vi "Read UI Refnum.vi"(8 "error in (no error)":errorcluster, 11 "SerializableObject in":refnum<class "SerializableObject.lvclass">) -> (0 "error out":errorcluster, 2 "VI Refnum":refnum<vi>, 3 "SerializableObject out":refnum<class "SerializableObject.lvclass">)   [LabVIEW 2015, in "SerializableObject.lvclass"]
uses:
  SerializableObject.lvclass
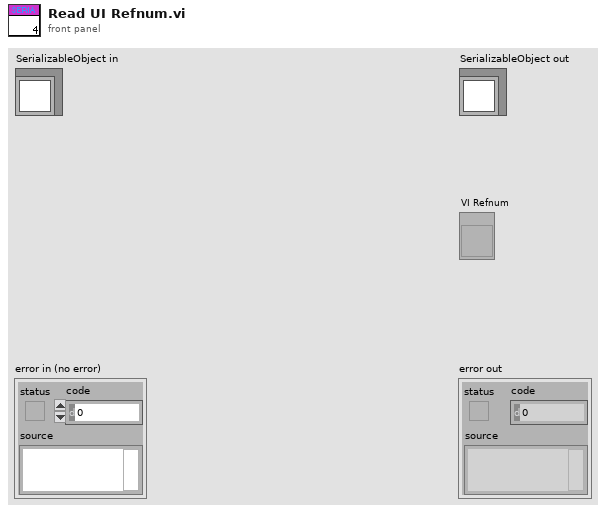
[diagram p1: front panel]
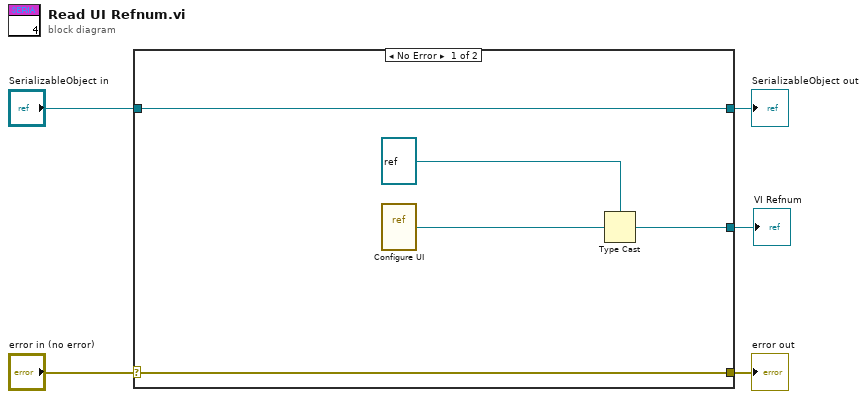
[diagram p0: block diagram]
diagram:
  n1 = case shown="No Error" "error in (no error)" {
    selector: "error in (no error)" -> [w9 w12]
    tunnel: [w9 w12] -> w4
    tunnel: [w10 w11] -> w2
    tunnel: "SerializableObject in" -> [w10 w11]
    tunnel: [w6 _] -> w1
    frame No Error {
      n2 = vi-ref "Configure UI.vi"() -> (w8:refnum<vi>)
      n3 = Type Cast(type=refnum<vi> refnum ("vi reference"), x=w8) -> (*(type *) &x=w6:refnum<vi>)
    }
    frame Error {
    }
  }
  "error out" <- w4
  "SerializableObject out" <- w2
  "VI Refnum" <- w1
